vi "UA_StringToCertificationsFiles.vi"(1 "Cerfitications String":string) -> (0 "file":path[](array[path]))   [LabVIEW 2013, in "CreateOPCUAServerAuto.lvlib"]
uses:
  CreateOPCUAServerAuto.lvlib
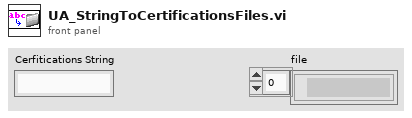
[diagram p1: front panel]
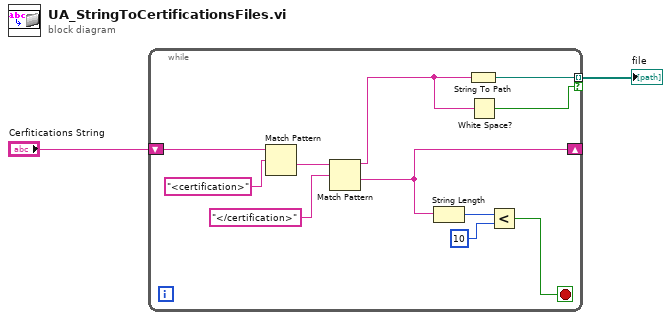
[diagram p0: block diagram]
diagram:
  n1 = while {
    shift-right: [w9] -> _
    shift-left: "Cerfitications String" -> [w13]
    tunnel: [w5] -> w1 mode=indexing if=w3
    stop <- w6 stop-if-true
    n2 = Match Pattern(string=w13, regular expression="<certification>") -> (after substring=w11:string)  [unwired: 1 in, 3 out]
    n3 = Match Pattern(string=w11, regular expression="</certification>") -> (before substring=w4:string, after substring=w9:string)  [unwired: 1 in, 2 out]
    n4 = String Length(string=w9) -> (length=w8:i32)
    n5 = String To Path(string=w4) -> (path=w5:path)
    n6 = White Space?(1:w4) -> (0:w3:bool)
    n7 = Less?(x=w8, y=10) -> (x < y?=w6:bool)
  }
  "file" <- w1
